vi "LVProjectShortcut_Provider_OnCommand.vi"(10 "Command ID":string, 11 "objects":T1[](array[typedef])) -> ()   [LabVIEW 2017]
uses:
  <resource>/Framework/Providers/API/ItemRef.ctl
panel:
  out "error out":errorcluster
  in  "error in":errorcluster
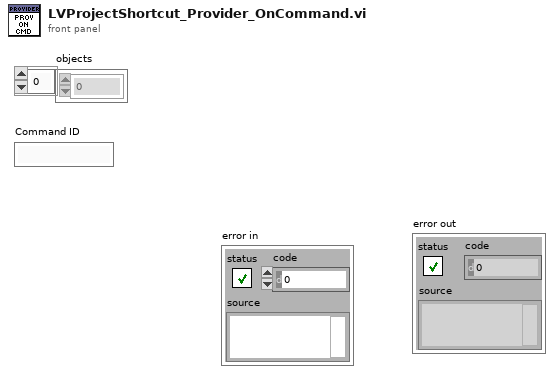
[diagram p1: front panel]
types:
  T1 = typedef "ItemRef.ctl" = u64
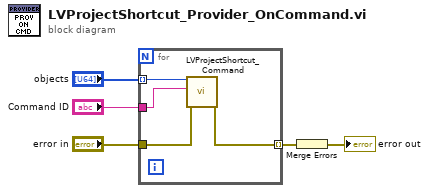
[diagram p0: block diagram]
diagram:
  n1 = for {
    tunnel: "objects" -> [w9] mode=indexing
    tunnel: "Command ID" -> [w8]
    tunnel: "error in" -> [w7]
    tunnel: [w6] -> w2 mode=indexing
    n2 = call <resource>:"LVProjectShortcut_Command.vi"("error in"=w7, "Command"=w8, "Object"=w9) -> ("error out"=w6:errorcluster)  [unwired: 8 in]
  }
  n3 = Merge Errors(w2) -> (→"error out":errorcluster)
